vi "4.2.WiFi Thingspeak_SmartConfig.vi"   [LabVIEW 2014]
uses:
  <vilib>/Aledyne-TSXperts/Arduino Compatible Compiler for LabVIEW/Code Generator/Arduino APIs/Digital/PinDirection.ctl
  <vilib>/Aledyne-TSXperts/Arduino Compatible Compiler for LabVIEW/addons/QwaveSys_ESP8266/QwaveSys_ESP8266.lvlib
  <vilib>/Aledyne-TSXperts/Arduino Compatible Compiler for LabVIEW/Arduino Compatible Compiler for LabVIEW.lvlib
types:
  T1 = typedef "Arduino Compatible Compiler for LabVIEW.lvlib/PinDirection.ctl" = enum16{" INPUT", "OUTPUT", " INPUT_PULLUP"}
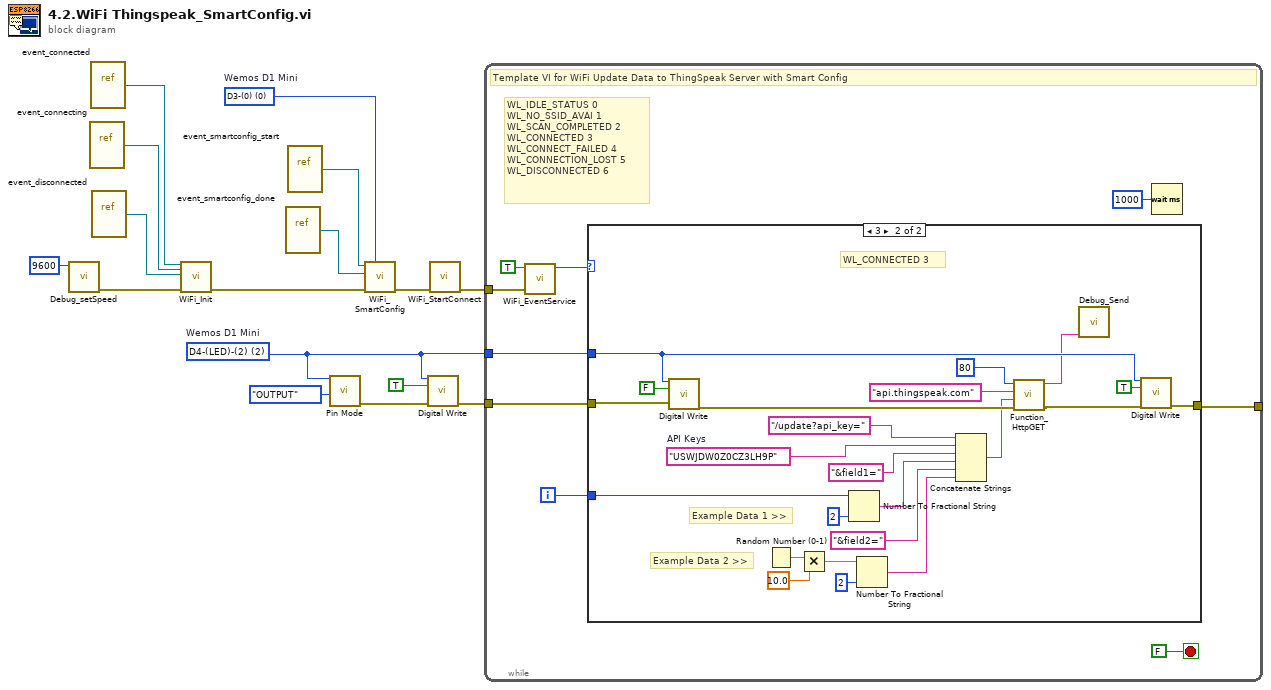
[diagram p0: block diagram]
diagram:
  w2 = u8 2 items=["D0-(16)"=16, "D1-SCL(5)"=5, "D2-SDA(4)"=4, "D3-(0)"=0, "D4-(LED)-(2)"=2, "D5-SCK(14)"=14, "D6-MISO(12)"=12, "D7-MOSI(13)"=13, "D8-SS(15)"=15, "TX(3)"=3, "RX(1)"=1, "ADC0,(17)"=17]  # Wemos D1 Mini
  w1 = u8 0 items=["D0-(16)"=16, "D1-SCL(5)"=5, "D2-SDA(4)"=4, "D3-(0)"=0, "D4-(LED)-(2)"=2, "D5-SCK(14)"=14, "D6-MISO(12)"=12, "D7-MOSI(13)"=13, "D8-SS(15)"=15, "TX(3)"=3, "RX(1)"=1, "ADC0,(17)"=17]  # Wemos D1 Mini
  n1 = call <vilib>:"Debug_setSpeed.vi"("Speed"=u32 9600) -> ("error out"=w8:errorcluster)  [unwired: 10 in]
  n2 = vi-ref "event_connecting.vi"() -> (w13:refnum<vi>)
  n3 = vi-ref "event_connected.vi"() -> (w12:refnum<vi>)
  n4 = vi-ref "event_disconnected.vi"() -> (w11:refnum<vi>)
  n5 = call <vilib>:"WiFi_Init.vi"("connected"=w12, "connecting"=w13, "disconnected"=w11, "error in (no error)"=w8) -> ("error out"=w16:errorcluster)  [unwired: 11 in]
  n6 = vi-ref "event_smartconfig_done.vi"() -> (w9:refnum<vi>)
  n7 = vi-ref "event_smartconfig_start.vi"() -> (w10:refnum<vi>)
  n8 = call <vilib>:"Pin Mode.vi"("pin"=w2, "direction"=PinDirection."OUTPUT") -> ("error out"=w5:errorcluster)  [unwired: 13 in]
  n9 = call <vilib>:"WiFi_SmartConfig.vi"("Smart Config Enter Pin"=w1, "error in (no error)"=w16, "smartconfig_done"=w9, "smartconfig_start"=w10) -> ("error out"=w15:errorcluster)  [unwired: 7 in]
  n10 = call <vilib>:"Digital Write.vi"("pin"=w2, "state"=TRUE, "error in (no error)"=w5) -> ("error out"=w3:errorcluster)  [unwired: 12 in]
  n11 = call <vilib>:"WiFi_StartConnect.vi"("error in (no error)"=w15) -> ("error out"=w14:errorcluster)  [unwired: 10 in]
  n12 = while {
    tunnel: w14 -> [w24]
    tunnel: w3 -> [w20]
    tunnel: w2 -> [w19]
    tunnel: [w17] -> _
    i -> [w18]
    stop <- FALSE stop-if-true
    # "WL_IDLE_STATUS\t0\nWL_NO_SSID_AVAI\t1\nWL_SCAN_COMPLETED\t2\nWL_CONNECTED\t3\nWL_CONNECT_FAILED\t4\nWL_CONNECTION_LOST\t5\nWL_DISCONNECTED\t6"
    # "Template VI for WiFi Update Data to ThingSpeak Server with Smart Config"
    n13 = call <vilib>:"WiFi_EventService.vi"("error in (no error)"=w24, "wait for connected (True)"=TRUE) -> ("Status"=w21:u16)  [unwired: 8 in, 1 out]
    n14 = case shown="3" w21 {
      tunnel: w20 -> [w26 w33]
      tunnel: w19 -> [_ w31]
      tunnel: w18 -> [_ w30]
      tunnel: [w26 w29] -> w17
      frame 0, Default {
        # "DISCONNECTED or default status"
      }
      frame 3 {
        w35 = "USWJDW0Z0CZ3LH9P"  # API Keys
        # "Example Data 2 >>"
        # "Example Data 1 >>"
        # "WL_CONNECTED\t3"
        n15 = call <vilib>:"Digital Write.vi"("pin"=w31, "state"=FALSE, "error in (no error)"=w33) -> ("error out"=w46:errorcluster)  [unwired: 12 in]
        n16 = Random Number (0-1)() -> (number: 0 to 1=w42:dbl)
        n17 = Multiply(x=w42, y=10.0) -> (x*y=w43:dbl)
        n18 = Number To Fractional String(number=w30, precision (6)=i16 2) -> (F-format string=w39:string)  [unwired: 2 in]
        n19 = Number To Fractional String(number=w43, precision (6)=i16 2) -> (F-format string=w45:string)  [unwired: 2 in]
        n20 = Concatenate Strings("/update?api_key=", w35, "&field1=", w39, "&field2=", w45) -> (w36:string)
        n21 = call <vilib>:"Function_HttpGET.vi"("error in (no error)"=w46, "URI"=w36, "Host"="api.thingspeak.com", "Port"=i8 80) -> ("error out"=w28:errorcluster, "Results"=w27:string)  [unwired: 6 in]
        n22 = call <vilib>:"Debug_Send.vi"("DATA"=w27) -> ()  [unwired: 11 in]
        n23 = call <vilib>:"Digital Write.vi"("pin"=w31, "state"=TRUE, "error in (no error)"=w28) -> ("error out"=w29:errorcluster)  [unwired: 12 in]
      }
    }
    n24 = Wait (ms)(milliseconds to wait=u32 1000) -> ()  [unwired: 1 out]
  }
